vi "Destroy Stop Event.vi"(8 "error in (no error)":errorcluster, 11 "Stop Event":refnum<user-event>) -> (0 "error out":errorcluster)   [LabVIEW 2016, in "Stop Event.lvlib"]
uses:
  Stop Event.lvlib
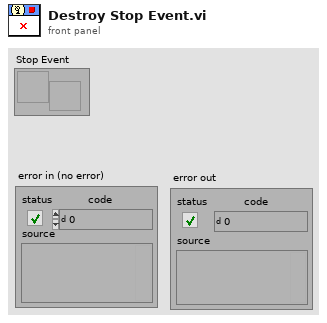
[diagram p1: front panel]
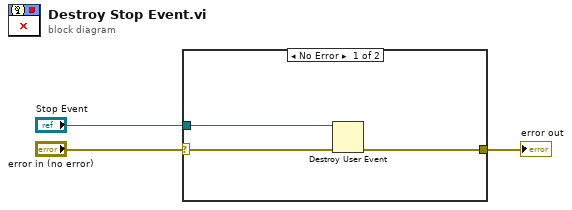
[diagram p0: block diagram]
diagram:
  n1 = case shown="No Error" "error in (no error)" {
    selector: "error in (no error)" -> [w6 w7]
    tunnel: [w4 w7] -> w2
    tunnel: "Stop Event" -> [w5 _]
    frame No Error {
      n2 = Destroy User Event(user event=w5, error in=w6) -> (error out=w4:errorcluster)
    }
    frame Error {
    }
  }
  "error out" <- w2
